vi "UpdateCrvsGraphIndex.vi"(8 "error in (no error)":errorcluster caption="entrée d'erreur (pas d'erreur)", 9 "DelGraphIndex":i32, 10 "CurvesParams":T1[](array[typedef]), 11 "XYGraphCurves":cluster{"Tableau":i32[]}[](array[cluster])) -> (0 "error out":errorcluster caption="sortie d'erreur", 2 "CurvesParams Out":T1[](array[typedef]), 3 "XYGraphCrvsOut":cluster{"Tableau":i32[]}[](array[cluster]))   [LabVIEW 2019, in "Interface.lvclass"]
uses:
  Interface.lvclass
  CurveSetup.ctl
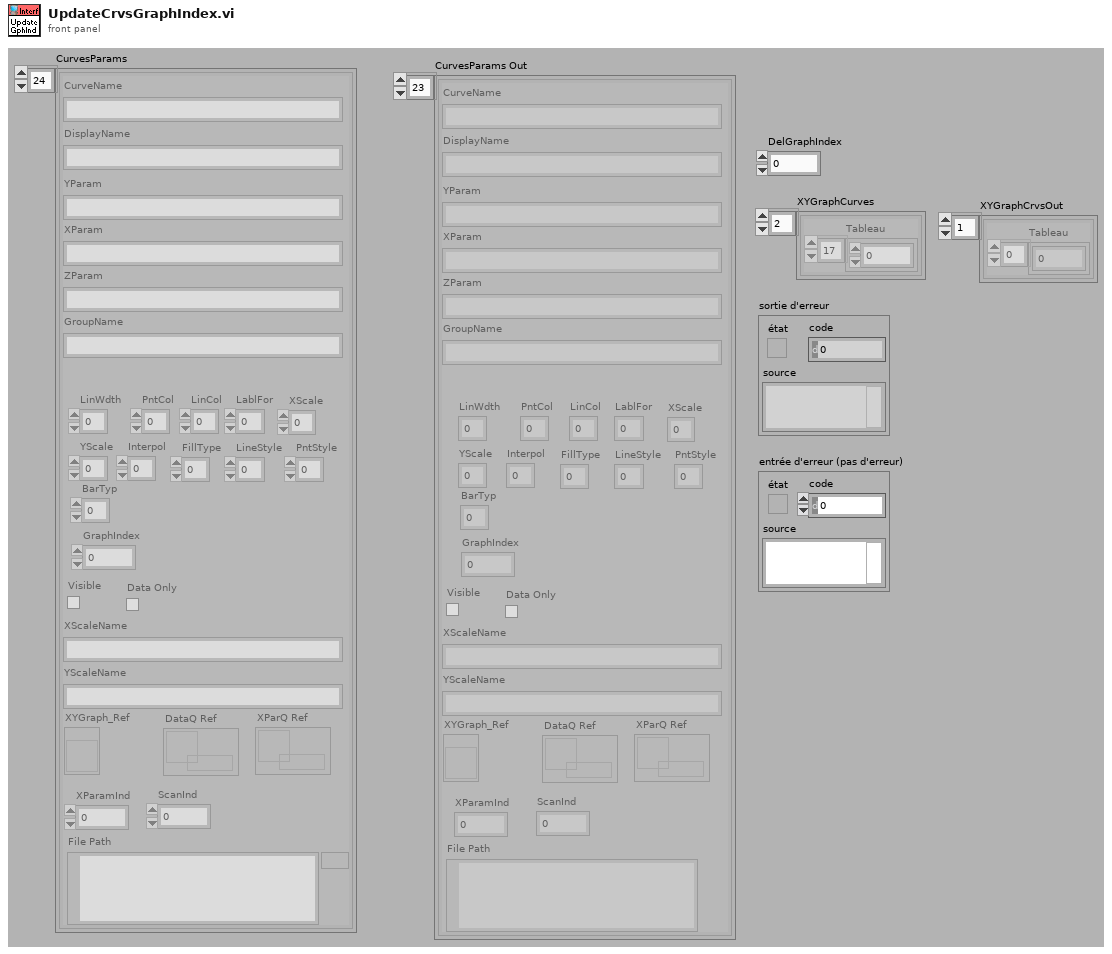
[diagram p1: front panel]
types:
  T1 = typedef "Interface.lvclass/CurveSetup.ctl" = cluster{"CurveName":string, "YParam":string, "XParam":string, "ZParam ":string, "GroupName":string, "LinWdth":u8, "PntCol":u32, "LinCol":u32, "LablFor":u8, "XScale":u32, "YScale":u32, "Interpol":u8, "DisplayName":string, "FillType":i16, "LineStyle":u8, "PntStyle":u8, "BarTyp":u8, "GraphIndex":i32, "Visible":bool, "XScaleName":string, "YScaleName":string, "XYGraph_Ref":refnum<vi>, "Data Only":bool, "DataQ Ref":refnum<queue>, "XParQ Ref":refnum<queue>, "XParamInd":i32, "ScanInd":i32, "File Path":path}
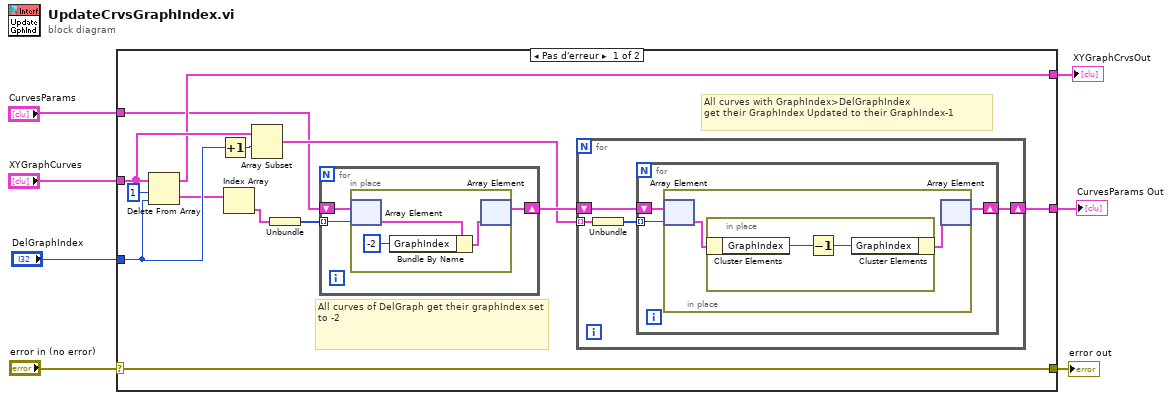
[diagram p0: block diagram]
diagram:
  n1 = case shown="Pas d'erreur" "error in (no error)" {
    selector: "error in (no error)" -> [w20 w38]
    tunnel: [w20 w38] -> w6
    tunnel: "CurvesParams" -> [w9 _]
    tunnel: "XYGraphCurves" -> [w16 _]
    tunnel: "DelGraphIndex" -> [w18 _]
    tunnel: [w15 _] -> w3
    tunnel: [w8 _] -> w1
    frame No Error {
      # "All curves with GraphIndex>DelGraphIndex\nget their GraphIndex Updated to their GraphIndex-1"
      # "All curves of DelGraph get their graphIndex set to -2"
      n2 = Delete From Array(array=w16, length=1 ("longueur"), index=w18) -> (deleted portion=w17:cluster{"Tableau":i32[]}[], array with subset deleted=w15:cluster{"Tableau":i32[]}[])
      n3 = Increment(x=w18) -> (x+1=w12:i32)
      n4 = Index Array(array=w17) -> (element=w13:cluster{"Tableau":i32[]})  [unwired: 1 in]
      n5 = Array Subset(array=w16, index=w12) -> (w10:cluster{"Tableau":i32[]}[])  [unwired: 1 in]
      n6 = Unbundle(w13) -> ("Tableau"=w14:i32[])
      n7 = for {
        tunnel: w14 -> [w34] mode=indexing
        shift-right: [w33] -> w11
        shift-left: w9 -> [w32]
        n8 = in-place {
          n9 = in-place-array #1(w32, w34) -> (w36:T1)
          n10 = Bundle By Name(cluster=w36, "GraphIndex"=-2) -> (w35:T1)
          n11 = in-place-array #1(w35) -> (w33:T1[])  [unwired: 1 out]
        }
      }
      n12 = for {
        tunnel: w10 -> [w23] mode=indexing
        shift-right: [w21] -> w8
        shift-left: w11 -> [w24]
        n13 = Unbundle(w23) -> ("Tableau"=w22:i32[])
        n14 = for {
          tunnel: w22 -> [w26] mode=indexing
          shift-right: [w25] -> w21
          shift-left: w24 -> [w27]
          n15 = in-place {
            n16 = in-place-array #2(w27, w26) -> (w29:T1)
            n17 = in-place {
              n18 = in-place-cluster #3(w29) -> ("GraphIndex"=w31:i32)
              n19 = Decrement(x=w31) -> (x-1=w30:i32)
              n20 = in-place-cluster #3("GraphIndex"=w30) -> (w28:T1)
            }
            n21 = in-place-array #2(w28) -> (w25:T1[])  [unwired: 1 out]
          }
        }
      }
    }
    frame Error {
    }
  }
  "error out" <- w6
  "XYGraphCrvsOut" <- w3
  "CurvesParams Out" <- w1
